vi "PH_Sixpack.get Information.vi"(0 "i ref in":refnum<vi>, 5 "error in":errorcluster) -> (14 "i ref out":refnum<vi>, 19 "error out":errorcluster)   [LabVIEW 2014, in "PH_Sixpack.lvlib"]
doc: "This VI queries information of the hardware, stores it to own attributes and puslihes it at DIM."
uses:
  PH_Sixpack.lvlib
  PH_Sixpack.Input.ctl
  PH_Stepmotor_BaseClass/PH_Stepmotor_BaseClass.Axis Activity.ctl
  instr.lib/SixPack/Sixpack - Driver.lvlib
  PH_Stepmotor_BaseClass/PH_Stepmotor_BaseClass.lvlib
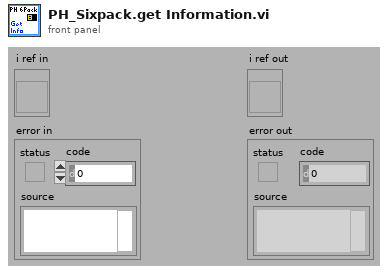
[diagram p1: front panel]
types:
  T1 = typedef "PH_Sixpack.lvlib/PH_Sixpack.Input.ctl" = cluster{"AnalogueValue (V)":dbl, "RefInput":bool}
  T2 = typedef "PH_Sixpack.lvlib/PH_Sixpack.Status.ctl" = enum32{"None", "Init", "Configure", "configured", "Close", "closed"}
  T3 = typedef "PH_Stepmotor_BaseClass.lvlib/PH_Stepmotor_BaseClass.Axis Activity.ctl" = enum16{"No Information", "stopped", "running", "Failure", "Alarm", "stopped at backward ES", "stopped at foreward ES"}
  T4 = typedef "PH_Stepmotor_BaseClass.lvlib/PH_Stepmotor_BaseClass.Axis Attributes.ctl" = cluster{"Settings":T5, "Endswitch?":bool, "DIM Service IDs":T7, "Activity":T3, "Configured?":bool, "Position":cluster{"Current":i32, "Target":i32}, "Position to set":cluster{"New?":bool, "Wanted":i32}, "Stop?":bool, "Reset?":bool, "Move?":bool, "Nothing connected?":bool}
  T5 = typedef "PH_Stepmotor_BaseClass.lvlib/PH_Stepmotor_BaseClass.Axis Settings.ctl" = cluster{"Sign change":bool, "Width":dbl, "Calibration":dbl, "Unit":string, "Motor Type":T6, "Unit Width":string, "Unit CF":string}
  T6 = typedef "PH_Stepmotor_BaseClass.lvlib/PH_Stepmotor_BaseClass.Motor Type.ctl" = enum16{"Unspecific", "OWIS 49.120.2633", "OWIS 49.060.1033", "OWIS 43.040.2558", "Diamond Motion 2200 series", "OWIS 49.120.266B.MV6", "Calorimeter", "Linear Stage 1", "MICOS VT-80", "MICOS VT-80 S", "Standa Rotstage nt0.95A", "PUF RA 320.200", "PUF RA 800.200", "PUF RA 800.400", "PUF RA 400.50", "1324.nn.800.50", "1324.n9c.800.50", "1324.nn.320.200", "1324.nn.400.200", "1324.nn.800.200", "1324.nn.400.50", "1324.8c9c.800.50", "1324.8c9c.400.200"}
  T7 = typedef "PH_Stepmotor_BaseClass.lvlib/PH_Stepmotor_BaseClass.Axis DIM Service IDs.ctl" = cluster{"Settings":i32, "Information":i32}
  T8 = typedef "Sixpack - Driver.lvlib/Activity.ctl" = enum16{"Inactive", "Ramp", "PI-Controller", "Rotation", "ReferenceSearch", "Reference Search", "MechanicalReference"}
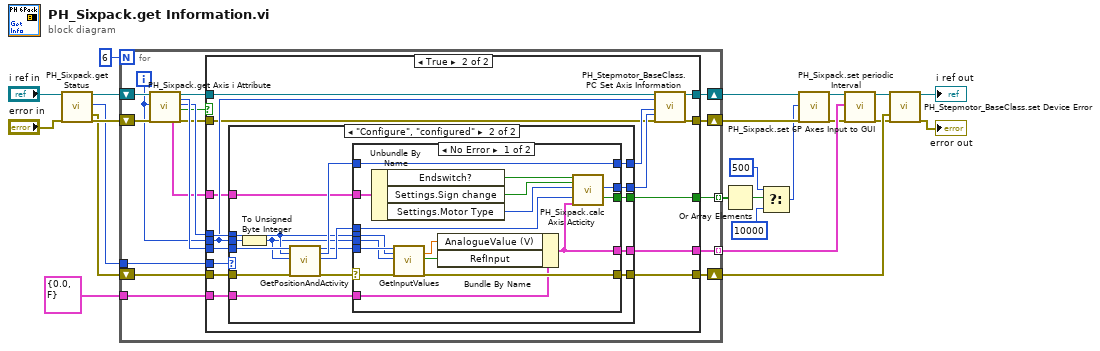
[diagram p0: block diagram]
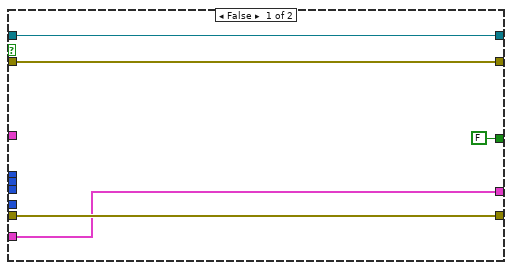
[diagram p2: hidden frame]
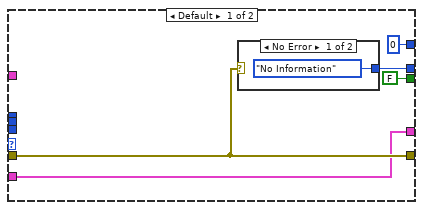
[diagram p3: hidden frame]
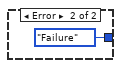
[diagram p4: hidden frame]
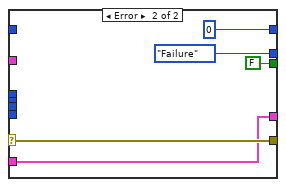
[diagram p5: hidden frame]
diagram:
  n1 = call "PH_Sixpack.get Status.vi"("VI in"="i ref in", "error in (no error)"="error in") -> ("VI out"=w20:refnum<vi>, "Status"=w17:T2, "Device Error"=w16:errorcluster, "error out"=w18:errorcluster)  [unwired: 14 in]
  n2 = for {
    N: 6 -> [_]
    shift-right: [w38] -> w15
    shift-left: w16 -> [w37]
    shift-right: [w33] -> w7
    shift-left: w20 -> [w36]
    shift-right: [w31] -> w14
    shift-left: w18 -> [w35]
    tunnel: w17 -> [w28]
    tunnel: [w27] -> w22 mode=indexing
    tunnel: T1 {"AnalogueValue (V)"=0.0, "RefInput"=FALSE} ("Input") -> [w26]
    tunnel: [w24] -> w5 mode=indexing
    i -> [w30]
    n3 = call "PH_Sixpack.get Axis i Attribute.vi"("VI in"=w36, "Axis"=w30, "error in"=w35) -> ("Axis Base Class Attributes"=w25:T4, "VI out"=w34:refnum<vi>, "HANDLE"=w40:i32, "SixPack ID(0)"=w39:u16, "Axis found?"=w29:bool, "error out"=w32:errorcluster)  [unwired: 10 in, 1 out]
    n4 = case shown="True" w29 {
      tunnel: w40 -> [_ w61]
      tunnel: w39 -> [_ w60]
      tunnel: [w43 w54] -> w38
      tunnel: w37 -> [w43 w59]
      tunnel: w34 -> [w45 w48]
      tunnel: [w45 w51] -> w33
      tunnel: w32 -> [w44 w47]
      tunnel: [w44 w52] -> w31
      tunnel: w30 -> [_ w55]
      tunnel: w28 -> [_ w58]
      tunnel: [w42 w53] -> w27
      tunnel: w26 -> [w42 w50]
      tunnel: w25 -> [_ w49]
      tunnel: [FALSE ("Running") w46] -> w24
      frame False {
      }
      frame True {
        n5 = case shown="\"Configure\", \"configured\"" w58 {
          tunnel: w61 -> [_ w84]
          tunnel: w60 -> [_ w72]
          tunnel: [w64 w76] -> w54
          tunnel: w59 -> [w64 w83]
          tunnel: [0 ("CurrentPosition") w80] -> w57
          tunnel: w55 -> [_ w79]
          tunnel: [w65 w82] -> w56
          tunnel: [w63 w74] -> w53
          tunnel: w50 -> [w63 w75]
          tunnel: w49 -> [_ w70]
          tunnel: [FALSE ("Running") w69] -> w46
          frame Default {
            n6 = case shown="No Error" w64 {
              tunnel: [PH_Stepmotor_BaseClass.Axis_Activity."No Information" ("Axis Activity") PH_Stepmotor_BaseClass.Axis_Activity."Failure" ("Axis Activity")] -> w65
              frame No Error {
              }
              frame Error {
              }
            }
          }
          frame "Configure", "configured" {
            n7 = To Unsigned Byte Integer(number=w79) -> (unsigned 8bit integer=w71:u8)
            n8 = call "GetPositionAndActivity.vi"("handle in"=w84, "UnitAddress(0)"=w72, "MotNr(0)"=w71, "error in"=w83) -> ("handle out"=w73:i32, "CurrentPosition"=w78:i32, "CurrentActivity"=w81:T8, "error out"=w77:errorcluster)  [unwired: 11 in, 1 out]
            n9 = case shown="No Error" w77 {
              selector: w77 -> [w98 w104]
              tunnel: [w100 PH_Stepmotor_BaseClass.Axis_Activity."Failure" ("Axis Activity")] -> w82
              tunnel: w81 -> [w101 _]
              tunnel: w78 -> [w99 _]
              tunnel: [w99 0 ("CurrentPosition")] -> w80
              tunnel: w70 -> [w90 _]
              tunnel: [w97 w104] -> w76
              tunnel: w75 -> [w91 w103]
              tunnel: [w86 w103] -> w74
              tunnel: w73 -> [w96 _]
              tunnel: w72 -> [w95 _]
              tunnel: w71 -> [w94 _]
              tunnel: [w85 FALSE ("Running")] -> w69
              frame No Error {
                n10 = Unbundle By Name(w90) -> ("Endswitch?"=w89:bool, "Settings.Sign change"=w88:bool, "Settings.Motor Type"=w87:T6)
                n11 = call "GetInputValues.vi"("handle in"=w96, "UnitAddress(0)"=w95, "Channel(0)"=w94, "error in"=w98) -> ("AnalogueValue (V)"=w93:dbl, "RefInput"=w92:bool, "error out"=w97:errorcluster)  [unwired: 10 in, 3 out]
                n12 = Bundle By Name(cluster=w91, "AnalogueValue (V)"=w93, "RefInput"=w92) -> (w86:T1)
                n13 = call "PH_Sixpack.calc Axis Acticity.vi"("Endswitch?"=w89, "Sign change"=w88, "Motor Type"=w87, "CurrentActivity"=w101, "Input in"=w86) -> ("Axis Activity"=w100:T3, "Running"=w85:bool)  [unwired: 13 in]
              }
              frame Error {
              }
            }
          }
        }
        n14 = call "PH_Stepmotor_BaseClass.PC Set Axis Information.vi"("i ref in"=w48, "axis"=w55, "Current Position (Steps)"=w57, "Axis Activity"=w56, "error in (no error)"=w47) -> ("i ref out"=w51:refnum<vi>, "error out"=w52:errorcluster)  [unwired: 13 in]
      }
    }
  }
  n15 = Or Array Elements(Boolean array=w5) -> (logical OR=w4:bool)
  n16 = Select(t=500, s=w4, f=10000 ("PeriodicInterval [ms]")) -> (s? t:f=w1:i32)
  n17 = call "PH_Sixpack.set periodic Interval.vi"("VI in"=w7, "PeriodicInterval [ms]"=w1, "error in (no error)"=w14) -> ("VI out"=w6:refnum<vi>, "error out"=w8:errorcluster)  [unwired: 15 in]
  n18 = call "PH_Sixpack.set 6P Axes Input to GUI.vi"("VI in"=w6, "Inputs"=w22, "error in"=w8) -> ("VI out"=w13:refnum<vi>, "error out"=w12:errorcluster)  [unwired: 15 in]
  n19 = call "PH_Stepmotor_BaseClass.set Device Error.vi"("i ref in"=w13, "Device Error"=w15, "error in"=w12) -> ("i ref out"=→"i ref out":refnum<vi>, "error out"=→"error out":errorcluster)  [unwired: 15 in]
